vi "Database.Cache.CheckStatus.vi"(7 "Idx":i32, 8 "error in":errorcluster, 10 "Data in":T2) -> (0 "error out":errorcluster, 2 "Data out":T1)   [LabVIEW 2016]
doc: "Write test results (measurement values) to proda database\n\nWabco 2017 All right reserved\nAuthor: maciej.szupienko@wabco-auto.com"
uses:
  Cache/Cache.ProductComponent.Data.ctl
  Drivers/PLC/LowLevel/PLC.DataBlock.PCcheckstatus.ctl
  Tools/Translator/Translator.Message.ctl
  Tools/EventLog/EventLog.EventSource.ctl
  Tools/EventLog/EventLog.EventLevel.ctl
  Tools/EventLog/EventLog.New(array).vi
  Drivers/PLC/LowLevel/PLC.DataBlock.PLCcheckstatus.ctl
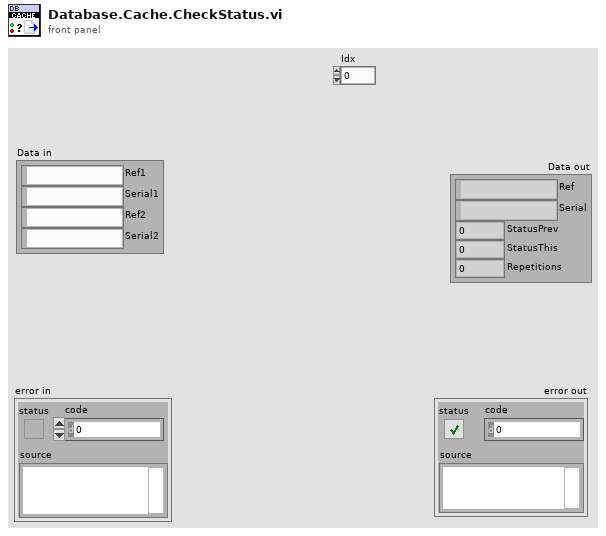
[diagram p1: front panel]
types:
  T1 = typedef "PLC.DataBlock.PCcheckstatus.ctl" = cluster{"Ref":string, "Serial":string, "StatusPrev":i8, "StatusThis":i8, "Repetitions":u8}
  T2 = typedef "PLC.DataBlock.PLCcheckstatus.ctl" = cluster{"Ref1":string, "Serial1":string, "Ref2":string, "Serial2":string}
  T3 = typedef "EventLog.EventSource.ctl" = enum16{"All", "Gui", "Cache", "PLC1", "PLC2", "PLC3", "DB", "DB01", "DB02", "DB03", "DB04", "DB05", "DB06", "DB07", "DB08", "DB09", "DB10", "DB11", "DB12", "DB13", "DB14", "DB15", "DB16"}
  T4 = typedef "Cache.ProductComponent.Data.ctl" = cluster{"Time":timestamp, "Station":string, "Ref1":string, "Serial1":string, "Ref2":string, "Serial2":string}
  T5 = typedef "Translator.Message.ctl" = enum16{"-", "Event confirmed", "Log out", "Log in", "Shutdown", "Cancel", "Start", "Continue", "Stop", "On", "Off", "OK", "NOK", "NOK %s", "This", "Prev", "Home", "Work", "In progress...", "Missing", "Empty", "Hardware failure", "Initial", "Error %d >> %s", "Error %d >> %s >> %s", "Starting %s", "Quitting %s", "Configured", "Initializing", "Quitting", "Loading", "Running %s", "Stopped", "Summary", "Do you want to continue?", "Do you want to exit?", "Log out?", "System", "All", "IDLE", "Translating...%s", "Not found", "Alarm %s", "Run", "Skip", "Abort", "Repeat", "Please wait...", "Database disconnected", "Login to database successful", "Login to database failed: %d; %s", "Get process step data for %s", "Changeover off", "Changeover into %s", "Product %s | %s found in cache with status %d at previous station", "Product %s | %s found in database with status %d at previous station", "Product %s | %s not found in cache at previous station", "Product %s | %s not found in database at previous station", "Product %s | %s found in cache with status %d at this station (%d repetion)", "Product %s | %s found in database with status %d at this station (%d repetition)", "Product %s | %s not found in cache at this station", "Product %s | %s not found in database at this station", "Product %s | %s found in cache for component %s | %s", "Product %s | %s found in database for component %s | %s", "Product not found in cache for component %s | %s", "Product not found in database for component %s | %s", "Product %s | %s connected with component %s | %s (cache)", "Product %s | %s connected with component %s | %s (database)", "New data for %s | %s (cache)", "New data for %s | %s (database)", "File %s moved (cache)", "File %s deleted (cache)", "Msg %d >> %s", "PLC LifeBit Failure", "Reconnecting DB", "Reconnecting PLC", "Free disk space is below 1GB - contact technician", "Unable to check product status", "Product %s SN %s checked in DB", "Unable To check status from station %s"}
  T6 = typedef "EventLog.EventLevel.ctl" = enum8{"Debug", "Info", "Warning", "Error"}
  T7 = cluster{"PrevStations":i32[], "ThisStations":i32[]}
  T8 = typedef "Cache.TestSteps.Fglb.ResultData.ctl" = cluster{"File":path, "Ref":string, "Serial":string, "Pr":T9, "PSr":T10, "TSr":cluster{"TSr":T11, "TVr":T12[]}[]}
  T9 = typedef "ProdaNG.ProcessResult.ctl" = cluster{"c_id":string, "productId":string, "processId":i32, "statusId":i32, "startTime":string, "endTime":string}
  T10 = typedef "ProdaNG.ProcessStepResult.ctl" = cluster{"c_id":string, "processResultId":string, "processStepId":i32, "statusId":i32, "operatorId":i32, "startTime":string, "endTime":string}
  T11 = typedef "ProdaNG.TestStepResult.ctl" = cluster{"c_id":string, "processStepResultId":string, "testStepId":i32, "statusId":i32}
  T12 = typedef "ProdaNG.TestValueResult.ctl" = cluster{"c_id":string, "testStepResultId":string, "testValueId":i32, "result":dbl, "statusId":i32, "contentId":string}
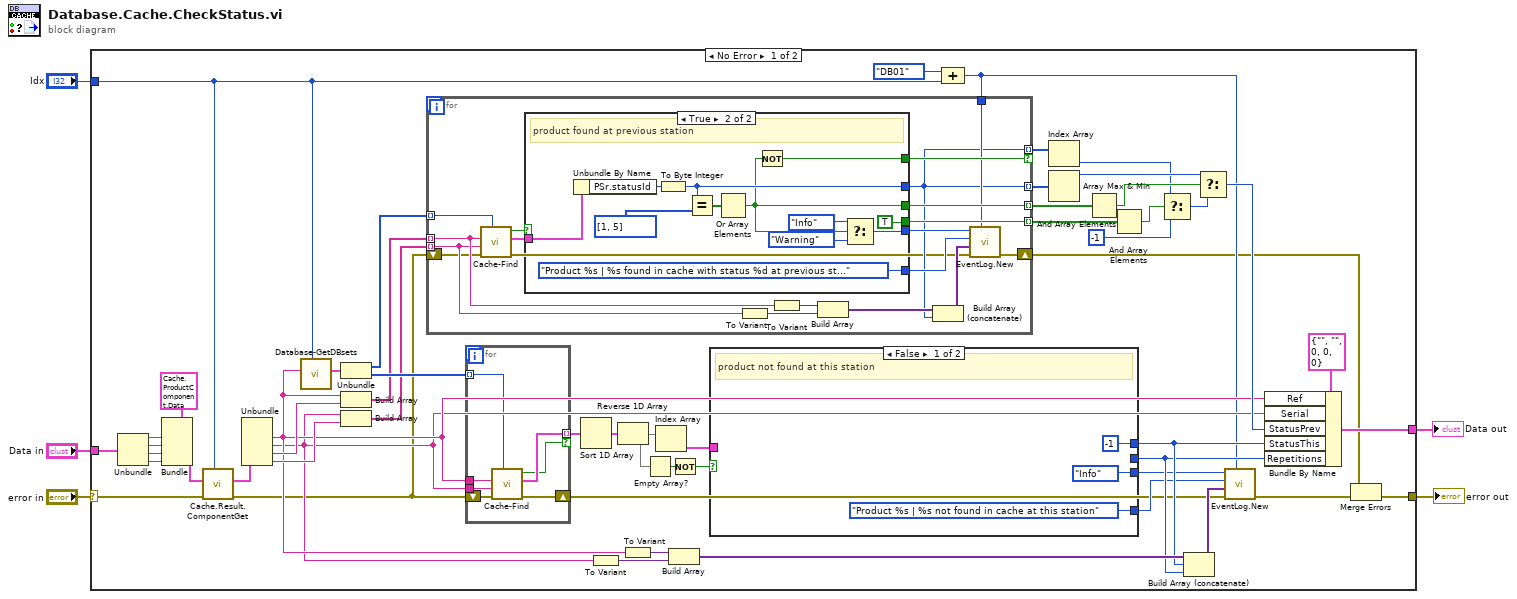
[diagram p0: block diagram]
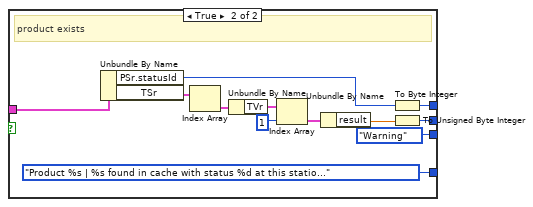
[diagram p2: hidden frame]
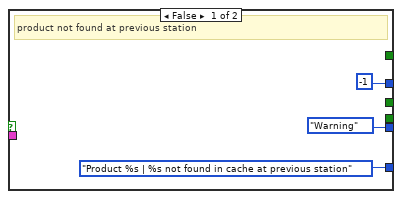
[diagram p3: hidden frame]
diagram:
  n1 = case shown="No Error" "error in" {
    selector: "error in" -> [w52 w115]
    tunnel: [w38 w115] -> w5
    tunnel: "Data in" -> [w51 _]
    tunnel: [w45 _] -> w2
    tunnel: "Idx" -> [w12 _]
    frame No Error {
      n2 = Unbundle(w51) -> ("Ref1"=w57:string, "Serial1"=w56:string, "Ref2"=w55:string, "Serial2"=w54:string)
      n3 = Bundle(cluster=T4 {"Time"=timestamp(0 s since 1904-01-01), "Station"="", "Ref1"="", "Serial1"="", "Ref2"="", "Serial2"=""} ("ProdComp in"), "Ref1"=w57, "Serial1"=w56, "Ref2"=w55, "Serial2"=w54) -> (w53:T4)  [unwired: 2 in]
      n4 = call "Cache.Result.ComponentGet.vi"("Idx"=w12, "error in (no error)"=w52, "ProdComp in"=w53) -> ("error out"=w11:errorcluster, "ProdComp out"=w10:T4)  [unwired: 6 in, 1 out]
      n5 = Unbundle(w10) -> ("Ref1"=w23:string, "Serial1"=w22:string, "Ref2"=w42:string, "Serial2"=w41:string)  [unwired: 2 out]
      n6 = call "Database-GetDBsets.vi"("Idx"=w12, "Variant"=w23) -> ("Variant Idx"=w9:T7)  [unwired: 5 in, 4 out]
      n7 = Unbundle(w9) -> ("PrevStations"=w44:i32[], "ThisStations"=w43:i32[])
      n8 = Build Array(w23, w42) -> (w40:string[])
      n9 = Build Array(w22, w41) -> (w39:string[])
      n10 = for {
        shift-right: [w61] -> w7
        shift-left: w11 -> [w65]
        tunnel: w43 -> [w62] mode=indexing
        tunnel: w23 -> [w64]
        tunnel: w22 -> [w63]
        tunnel: [w60] -> w48 mode=indexing if=w59
        n11 = call "Cache-Find.vi"("Idx"=w62, "error in"=w65, "Serial"=w63, "Variant"=w64) -> ("error out"=w61:errorcluster, "Result"=w60:T8, "Found"=w59:bool)  [unwired: 4 in, 1 out]
      }
      n12 = Sort 1D Array(array=w48) -> (sorted array=w50:T8[])
      n13 = To Variant(anything=w22) -> (Variant=w25:variant)
      n14 = Reverse 1D Array(array=w50) -> (reversed array=w47:T8[])
      n15 = To Variant(anything=w23) -> (Variant=w24:variant)
      n16 = Empty Array?(array=w47) -> (empty?=w26:bool)
      n17 = Index Array(array=w47) -> (element=w8:T8)  [unwired: 1 in]
      n18 = Build Array(w24, w25) -> (w21:variant[])
      n19 = Not(x=w26) -> (.not. x?=w49:bool)
      n20 = case shown="False" w49 {
        tunnel: w8 -> [_ w69]
        tunnel: [_ w75] -> w19
        tunnel: [i8 -1 w74] -> w20
        tunnel: [EventLog.EventLevel."Info" ("Level (Info)") EventLog.EventLevel."Warning" ("Level (Info)")] -> w14
        tunnel: [Translator.Message."Product %s | %s not found in cache at this station" ("Message (-)") Translator.Message."Product %s | %s found in cache with status %d at this station (%d repetion)" ("Message (-)")] -> w13
        frame False {
          # "product not found at this station"
        }
        frame True {
          # "product exists"
          n21 = Unbundle By Name(w69) -> ("PSr.statusId"=w73:i32, "TSr"=w80:cluster{"TSr":T11, "TVr":T12[]}[])
          n22 = Index Array(array=w80) -> (element=w79:cluster{"TSr":T11, "TVr":T12[]})  [unwired: 1 in]
          n23 = Unbundle By Name(w79) -> ("TVr"=w78:T12[])
          n24 = Index Array(array=w78, index=1) -> (element=w77:T12)
          n25 = Unbundle By Name(w77) -> ("result"=w76:dbl)
          n26 = To Byte Integer(number=w73) -> (8bit integer=w74:i8)
          n27 = To Unsigned Byte Integer(number=w76) -> (unsigned 8bit integer=w75:u8)
        }
      }
      n28 = Compound Arithmetic op=ADD(EventLog.EventSource."DB01" ("Source (All)"), w12) -> (w16:i32)
      n29 = for {
        shift-right: [w91] -> w15
        shift-left: w11 -> [w85]
        tunnel: w44 -> [w82] mode=indexing
        tunnel: w40 -> [w87] mode=indexing
        tunnel: w39 -> [w86] mode=indexing
        tunnel: [w88] -> w35 mode=indexing
        tunnel: [w99] -> w36 mode=indexing
        tunnel: [w98] -> w37 mode=indexing
        tunnel: [w88] -> w30 mode=indexing if=w97
        tunnel: w16 -> [w94]
        n30 = call "Cache-Find.vi"("Idx"=w82, "error in"=w85, "Serial"=w86, "Variant"=w87) -> ("error out"=w81:errorcluster, "Result"=w83:T8, "Found"=w84:bool)  [unwired: 4 in, 1 out]
        n31 = case shown="True" w84 {
          tunnel: [i8 -1 w110] -> w88
          tunnel: [_ TRUE] -> w99
          tunnel: [_ w107] -> w98
          tunnel: [_ w109] -> w97
          tunnel: [EventLog.EventLevel."Warning" ("Level (Info)") w104] -> w90
          tunnel: [Translator.Message."Product %s | %s not found in cache at previous station" ("Message (-)") Translator.Message."Product %s | %s found in cache with status %d at previous station" ("Message (-)")] -> w89
          tunnel: w83 -> [_ w103]
          frame False {
            # "product not found at previous station"
          }
          frame True {
            # "product found at previous station"
            n32 = Unbundle By Name(w103) -> ("PSr.statusId"=w114:i32)
            n33 = To Byte Integer(number=w114) -> (8bit integer=w110:i8)
            n34 = Equal?(x=w110, y=i8[] [1, 5]) -> (x = y?=w112:bool[])
            n35 = Or Array Elements(Boolean array=w112) -> (logical OR=w107:bool)
            n36 = Not(x=w107) -> (.not. x?=w109:bool)
            n37 = Select(t=EventLog.EventLevel."Info" ("Level (Info)"), s=w107, f=EventLog.EventLevel."Warning" ("Level (Info)")) -> (s? t:f=w104:T6)
          }
        }
        n38 = To Variant(anything=w86) -> (Variant=w96:variant)
        n39 = To Variant(anything=w87) -> (Variant=w95:variant)
        n40 = Build Array(w95, w96) -> (w93:variant[])
        n41 = Build Array (concatenate)(w93, w88) -> (w92:variant[])
        n42 = call-poly "EventLog.New.vi"("Source (All)"=w94, "error in (no error)"=w81, "Arguments"=w92, "Message (-)"=w89, "Level (Info)"=w90) -> ("error out"=w91:errorcluster)  [unwired: 5 in, 1 out]
      }
      n43 = Index Array(array=w30) -> (element=w29:i8)  [unwired: 1 in]
      n44 = Array Max & Min(array=w35) -> (max value=w34:i8)  [unwired: 3 out]
      n45 = And Array Elements(Boolean array=w37) -> (logical AND=w33:bool)
      n46 = And Array Elements(Boolean array=w36) -> (logical AND=w32:bool)
      n47 = Select(t=w29, s=w32, f=i8 -1 ("max value")) -> (s? t:f=w31:i8)
      n48 = Build Array (concatenate)(w21, w20, w19) -> (w18:variant[])
      n49 = Select(t=w34, s=w33, f=w31) -> (s? t:f=w28:i8)
      n50 = call-poly "EventLog.New.vi"("Source (All)"=w16, "error in (no error)"=w7, "Arguments"=w18, "Message (-)"=w13, "Level (Info)"=w14) -> ("error out"=w17:errorcluster)  [unwired: 5 in, 1 out]
      n51 = Bundle By Name(cluster=T1 {"Ref"="", "Serial"="", "StatusPrev"=0, "StatusThis"=0, "Repetitions"=0} ("Data out"), "Ref"=w23, "Serial"=w22, "StatusPrev"=w28, "StatusThis"=w20, "Repetitions"=w19) -> (w45:T1)
      n52 = Merge Errors(w15, w17) -> (w38:errorcluster)
    }
    frame Error {
    }
  }
  "error out" <- w5
  "Data out" <- w2
